vi "Main.vi"() -> ()   [LabVIEW 2013]
uses:
  <vilib>/Instr/_visa.llb/VISA Configure Serial Port (Instr).vi
panel:
  out "range finder output":string
  out "range [inches]":u32(slide) scale=0.0..80.0
  in  "[ESC]":bool
  # "Sonic Range Finder demo"
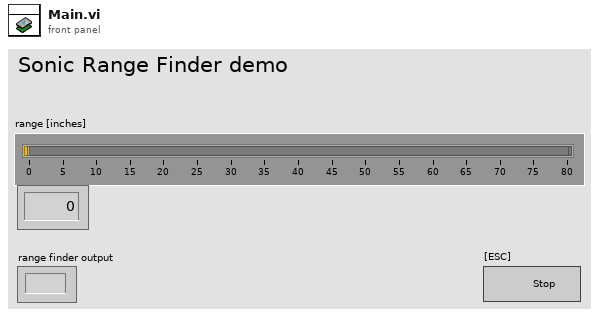
[diagram p1: front panel]
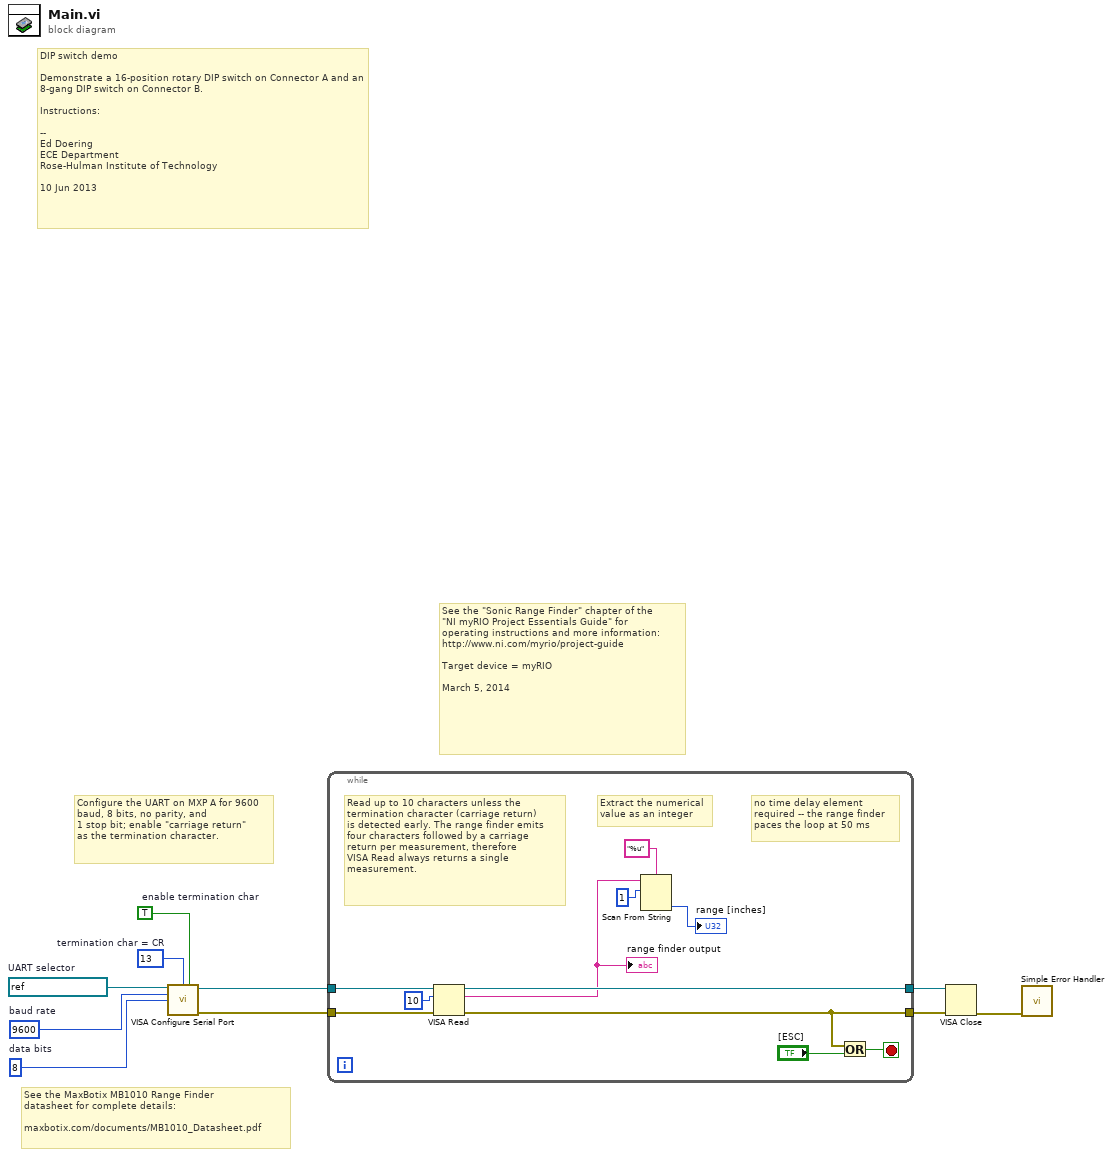
[diagram p0: block diagram]
diagram:
  w1 = u8 13  # termination char = CR
  w10 = refnum<visa-resource-name> "ASRL1::INSTR"  # UART selector
  w2 = TRUE  # enable termination char
  w3 = u16 8  # data bits
  w4 = u32 9600  # baud rate
  # "See the \"Sonic Range Finder\" chapter of the\n\"NI myRIO Project Essentials Guide\" for\noperating instructions and more information: \nhttp://www.ni.com/myrio/project-guide\n\nTarget device = myRIO\n\nMarch 5, 2014"
  # "See the MaxBotix MB1010 Range Finder\ndatasheet for complete details:\n\nmaxbotix.com/documents/MB1010_Datasheet.pdf"
  # "Configure the UART on MXP A for 9600 baud, 8 bits, no parity, and\n1 stop bit; enable \"carriage return\"\nas the termination character."
  # "DIP switch demo\n\nDemonstrate a 16-position rotary DIP switch on Connector A and an 8-gang DIP switch on Connector B.\n\nInstructions:\n\n-- \nEd Doering\nECE Department\nRose-Hulman Institute of Technology\n\n10 Jun 2013"
  n1 = call-poly "VISA Configure Serial Port"("VISA resource name"=w10, "termination char\n(0xA = '\\n' = LF)"=w1, "Enable Termination\nChar (T)"=w2, "baud rate (9600)"=w4, "data bits (8)"=w3) -> ("VISA resource name out"=w9:refnum<visa-resource-name>, "error out"=w8:errorcluster)  [unwired: 9 in]
  n2 = while {
    tunnel: w9 -> [w16]
    tunnel: w8 -> [w12]
    tunnel: [w14] -> w7
    tunnel: [w11] -> w6
    stop <- w21 stop-if-true
    # "Read up to 10 characters unless the \ntermination character (carriage return)\nis detected early. The range finder emits\nfour characters followed by a carriage\nreturn per measurement, therefore\nVISA Read always returns a single measurement."
    # "no time delay element\nrequired -- the range finder\npaces the loop at 50 ms"
    # "Extract the numerical\nvalue as an integer"
    n3 = VISA Read(VISA resource name=w16, byte count=u32 10, error in (no error)=w12) -> (VISA resource name out=w14:refnum<visa-resource-name>, read buffer=w13:string, error out=w11:errorcluster)  [unwired: 1 out]
    "range finder output" <- w13
    n4 = Scan From String "Scan From String"(format string="%u", input string=w13, initial scan location=u32 1) -> (output 1=→"range [inches]":u32)  [unwired: 2 in, 3 out]
    n5 = Or(x=w11, y="[ESC]") -> (x .or. y?=w21:bool)
  }
  n6 = VISA Close(VISA resource name=w7, error in (no error)=w6) -> (error out=w5:errorcluster)
  n7 = call <vilib>:"Simple Error Handler.vi"("error in (no error)"=w5) -> ()  [unwired: 4 in, 5 out]
